vi "Sort Transactions.vi"(10 "Transactions In":T2[](array[typedef])=[{"Dataset Source"=enum."LBCB 1", "Dataset Type"=enum."Displacement", "Hold"=TRUE, "Volts"=FALSE, "Tag"=""}, {"Dataset Source"=enum."LBCB 1", "Dataset Type"=enum."Force", "Hold"=TRUE, "Volts"=FALSE, "Tag"=""}, {"Dataset Source"=enum."LBCB 1", "Dataset Type"=enum."LVDT", "Hold"=TRUE, "Volts"=FALSE, "Tag"=""}, {"Dataset Source"=enum."LBCB 1", "Dataset Type"=enum."Load Cell", "Hold"=TRUE, "Volts"=FALSE, "Tag"=""}, {"Dataset Source"=enum."LBCB 2", "Dataset Type"=enum."Displacement", "Hold"=TRUE, "Volts"=FALSE, "Tag"=""}, {"Dataset Source"=enum."LBCB 2", "Dataset Type"=enum."Force", "Hold"=TRUE, "Volts"=FALSE, "Tag"=""}, {"Dataset Source"=enum."LBCB 2", "Dataset Type"=enum."LVDT", "Hold"=TRUE, "Volts"=FALSE, "Tag"=""}, {"Dataset Source"=enum."LBCB 2", "Dataset Type"=enum."Load Cell", "Hold"=TRUE, "Volts"=FALSE, "Tag"=""}, {"Dataset Source"=enum."Combined", "Dataset Type"=enum."Displacement", "Hold"=TRUE, "Volts"=FALSE, "Tag"=""}, {"Dataset Source"=enum."Combined", "Dataset Type"=enum."Force", "Hold"=TRUE, "Volts"=FALSE, "Tag"=""}, {"Dataset Source"=enum."LBCB 1", "Dataset Type"=enum."Actuator Command", "Hold"=FALSE, "Volts"=FALSE, "Tag"=""}, {"Dataset Source"=enum."LBCB 1", "Dataset Type"=enum."Displacement Command", "Hold"=FALSE, "Volts"=FALSE, "Tag"=""}, {"Dataset Source"=enum."LBCB 2", "Dataset Type"=enum."Actuator Command", "Hold"=FALSE, "Volts"=FALSE, "Tag"=""}, {"Dataset Source"=enum."LBCB 2", "Dataset Type"=enum."Displacement Command", "Hold"=FALSE, "Volts"=FALSE, "Tag"=""}, {"Dataset Source"=enum."Combined", "Dataset Type"=enum."Displacement Command", "Hold"=FALSE, "Volts"=FALSE, "Tag"=""}]) -> (2 "Transactions Out":T2[](array[typedef])=[{"Dataset Source"=enum."LBCB 1", "Dataset Type"=enum."Displacement", "Hold"=TRUE, "Volts"=FALSE, "Tag"=""}, {"Dataset Source"=enum."LBCB 1", "Dataset Type"=enum."Force", "Hold"=TRUE, "Volts"=FALSE, "Tag"=""}, {"Dataset Source"=enum."LBCB 1", "Dataset Type"=enum."LVDT", "Hold"=TRUE, "Volts"=FALSE, "Tag"=""}, {"Dataset Source"=enum."LBCB 1", "Dataset Type"=enum."Load Cell", "Hold"=TRUE, "Volts"=FALSE, "Tag"=""}, {"Dataset Source"=enum."LBCB 2", "Dataset Type"=enum."Displacement", "Hold"=TRUE, "Volts"=FALSE, "Tag"=""}, {"Dataset Source"=enum."LBCB 2", "Dataset Type"=enum."Force", "Hold"=TRUE, "Volts"=FALSE, "Tag"=""}, {"Dataset Source"=enum."LBCB 2", "Dataset Type"=enum."LVDT", "Hold"=TRUE, "Volts"=FALSE, "Tag"=""}, {"Dataset Source"=enum."LBCB 2", "Dataset Type"=enum."Load Cell", "Hold"=TRUE, "Volts"=FALSE, "Tag"=""}, {"Dataset Source"=enum."Combined", "Dataset Type"=enum."Displacement", "Hold"=TRUE, "Volts"=FALSE, "Tag"=""}, {"Dataset Source"=enum."Combined", "Dataset Type"=enum."Force", "Hold"=TRUE, "Volts"=FALSE, "Tag"=""}, {"Dataset Source"=enum."LBCB 1", "Dataset Type"=enum."Actuator Command", "Hold"=FALSE, "Volts"=FALSE, "Tag"=""}, {"Dataset Source"=enum."LBCB 1", "Dataset Type"=enum."Displacement Command", "Hold"=FALSE, "Volts"=FALSE, "Tag"=""}, {"Dataset Source"=enum."LBCB 2", "Dataset Type"=enum."Actuator Command", "Hold"=FALSE, "Volts"=FALSE, "Tag"=""}, {"Dataset Source"=enum."LBCB 2", "Dataset Type"=enum."Displacement Command", "Hold"=FALSE, "Volts"=FALSE, "Tag"=""}, {"Dataset Source"=enum."Combined", "Dataset Type"=enum."Displacement Command", "Hold"=FALSE, "Volts"=FALSE, "Tag"=""}])   [LabVIEW 2013]
uses:
  Dataset Transaction Id.ctl
  Dataset Source.ctl
  Dataset Type.ctl
  Apps/Yes No Button.ctl
panel:
  in  "Sorted Dateset Types":T1[](array[typedef])=[enum."Displacement Command", enum."Displacement", enum."Force", enum."Actuator Command", enum."LVDT", enum."Load Cell", enum."Servo Error"]
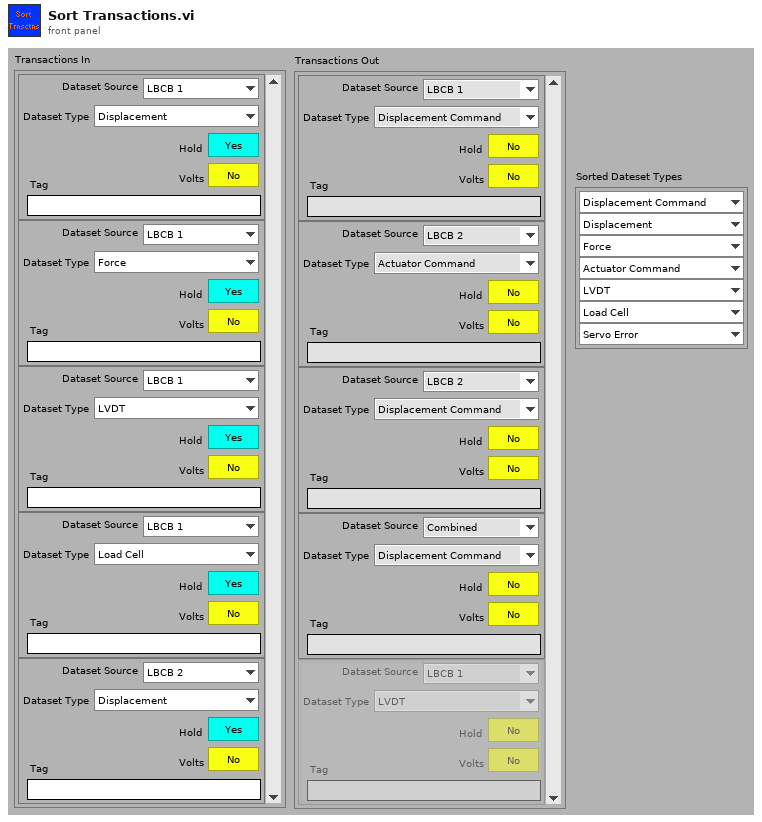
[diagram p1: front panel]
types:
  T1 = typedef "Dataset Type.ctl" = enum16{"LVDT", "Load Cell", "Actuator Command", "Servo Error", "Displacement Command", "Displacement", "Force"}
  T2 = typedef "Dataset Transaction Id.ctl" = cluster{"Dataset Source":T3, "Dataset Type":T1, "Hold":T4, "Volts":T4, "Tag":string}
  T3 = typedef "Dataset Source.ctl" = enum16{"LBCB 1", "LBCB 2", "Combined", "External Sensors"}
  T4 = typedef "Yes No Button.ctl" = bool
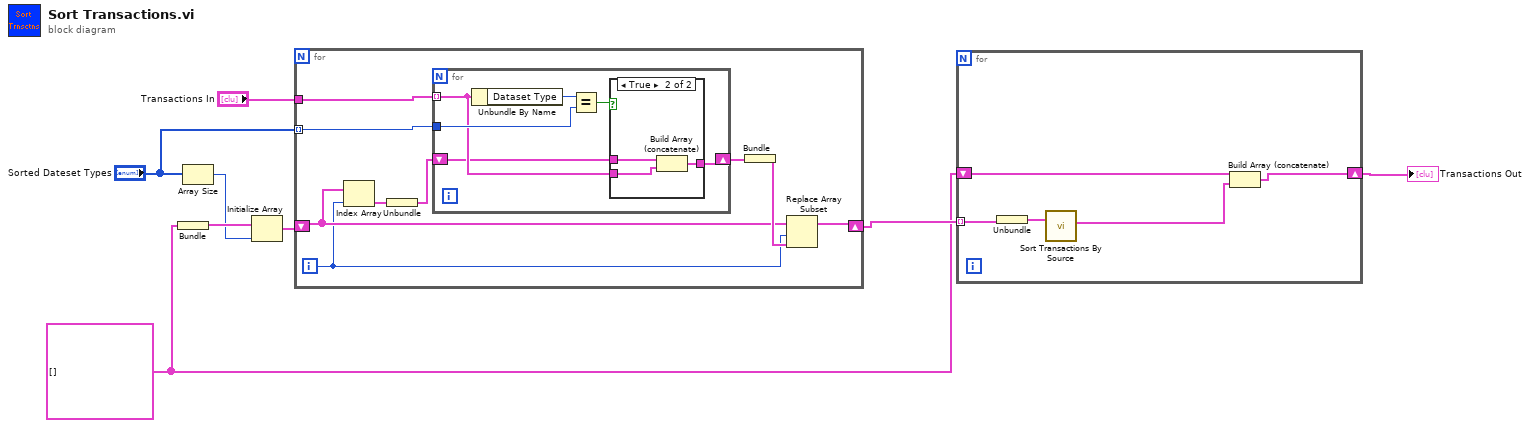
[diagram p0: block diagram]
diagram:
  w1 = T2[] []
  n1 = Bundle(w1) -> (w8:cluster{T2[]})  [unwired: 1 in]
  n2 = Array Size(array="Sorted Dateset Types") -> (size(s)=w7:i32)
  n3 = Initialize Array(w8, w7) -> (w6:cluster{T2[]}[])
  n4 = for {
    shift-right: [w13] -> w3
    shift-left: w6 -> [w12]
    tunnel: "Sorted Dateset Types" -> [w17] mode=indexing
    tunnel: "Transactions In" -> [w16]
    i -> [w11]
    n5 = Index Array(array=w12, index=w11) -> (element=w10:cluster{T2[]})
    n6 = Unbundle(w10) -> (w9:T2[])
    n7 = for {
      tunnel: w17 -> [w22]
      tunnel: w16 -> [w19] mode=indexing
      shift-right: [w20] -> w14
      shift-left: w9 -> [w18]
      n8 = Unbundle By Name(w19) -> ("Dataset Type"=w23:T1)
      n9 = Equal?(x=w23, y=w22) -> (x = y?=w21:bool)
      n10 = case shown="True" w21 {
        tunnel: [w24 w27] -> w20
        tunnel: w19 -> [_ w26]
        tunnel: w18 -> [w24 w25]
        frame False {
        }
        frame True {
          n11 = Build Array (concatenate)(w25, w26) -> (w27:T2[])
        }
      }
    }
    n12 = Bundle(w14) -> (w15:cluster{T2[]})  [unwired: 1 in]
    n13 = Replace Array Subset(array=w12, new element=w15, index=w11) -> (w13:cluster{T2[]}[])
  }
  n14 = for {
    tunnel: w3 -> [w32] mode=indexing
    shift-right: [w30] -> w2
    shift-left: w1 -> [w28]
    n15 = Unbundle(w32) -> (w31:T2[])
    n16 = call "Sort Transactions By Source.vi"("Transactions In"=w31) -> ("Transactions Out"=w29:T2[])  [unwired: 10 in]
    n17 = Build Array (concatenate)(w28, w29) -> (w30:T2[])
  }
  "Transactions Out" <- w2
